vi "TPNT_LogTP.vi"(6 "UTC":bool, 7 "tpnt_logfile":path, 8 "error in (no error)":errorcluster, 9 "tp separator":string=", ", 10 "Device":T1={"device"="", "devupdate"=0.0, "next_update"=0, "devinterface"="", "TPs"=[], "Alarms"=TRUE, "monitor"=TRUE, "log sep"=""} {"TPs"."Log"."updaterate" format="%.2f"; "TPs"."Samples"."Values" format="%.2f"; "TPs"."Samples"."samples" min=1 step=1; "TPs"."Limits"."Nominal" format="%.2f"; "TPs"."Limits"."Upper" format="%.2f"; "TPs"."Limits"."Lower" format="%.2f"; "TPs"."update_rate" format="%.2f"; "devupdate" format="%.2f"}) -> (0 "error out":errorcluster, 2 "Devices out":T1={"device"="", "devupdate"=0.0, "next_update"=0, "devinterface"="", "TPs"=[], "Alarms"=TRUE, "monitor"=TRUE, "log sep"=""} {"TPs"."Log"."updaterate" format="%.2f"; "TPs"."Samples"."Values" format="%.2f"; "TPs"."Samples"."samples" min=1 step=1; "TPs"."Limits"."Nominal" format="%.2f"; "TPs"."Limits"."Upper" format="%.2f"; "TPs"."Limits"."Lower" format="%.2f"; "TPs"."update_rate" format="%.2f"; "devupdate" format="%.2f"})   [LabVIEW 2016]
uses:
  TPNT_DeviceTPs.ctl
  TPNT_TP.ctl
  TPNT_Limits.ctl
  TPNT_Samples.ctl
  TPNT_Log.ctl
panel:
  in  "maxfilesize":u32=1024
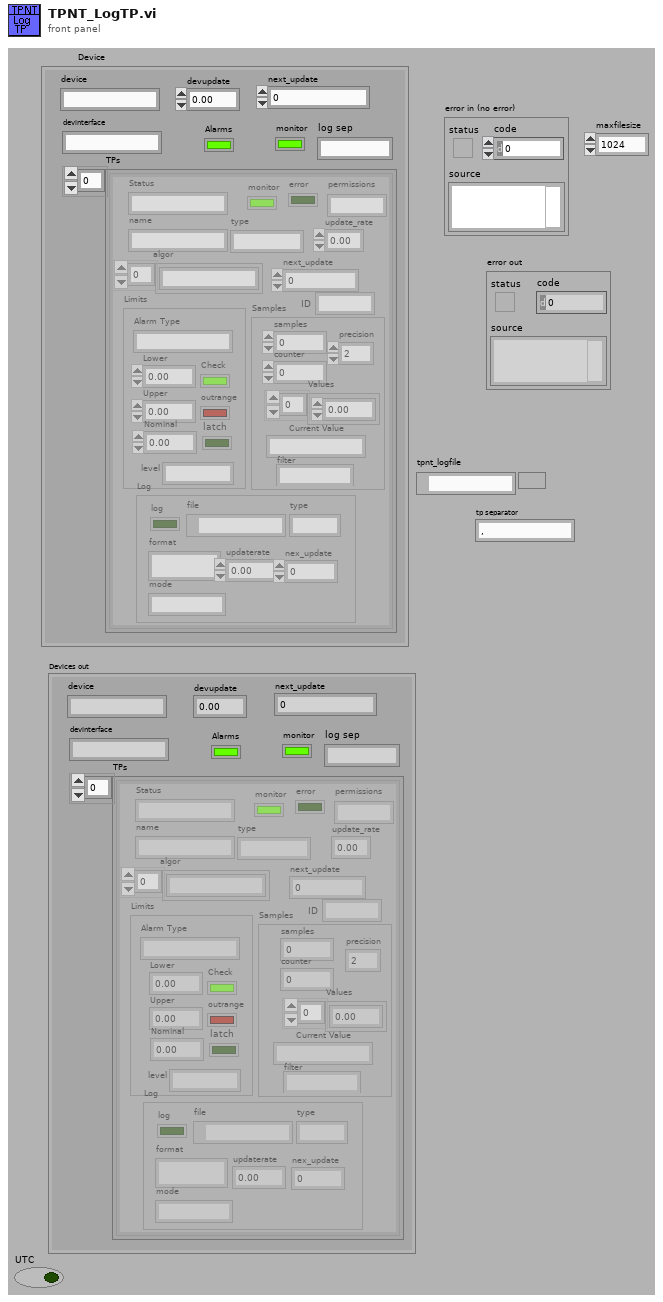
[diagram p1: front panel]
types:
  T1 = typedef "TPNT_DeviceTPs.ctl" = cluster{"device":string, "devupdate":dbl, "next_update":u32, "devinterface":string, "TPs":T2[], "Alarms":bool, "monitor":bool, "log sep":string}
  T2 = typedef "TPNT_TP.ctl" = cluster{"name":string, "type":string, "algor":string[], "update_rate":sgl, "Limits":T3, "Samples":T4, "next_update":u32, "Status":string, "monitor":bool, "error":bool, "Log":T5, "permissions":string, "ID":string}
  T3 = typedef "TPNT_Limits.ctl" = cluster{"Alarm Type":string, "Lower ":dbl, "Upper":dbl, "Nominal":dbl, "outrange":bool, "Check":bool, "latch":bool, "level":string}
  T4 = typedef "TPNT_Samples.ctl" = cluster{"samples":i32, "counter":i32, "Values":dbl[], "Current Value":string, "filter":string, "precision":u8}
  T5 = typedef "TPNT_Log.ctl" = cluster{"log":bool, "file":path, "type":string, "format":string, "updaterate":dbl, "nex_update":u32, "mode":string}
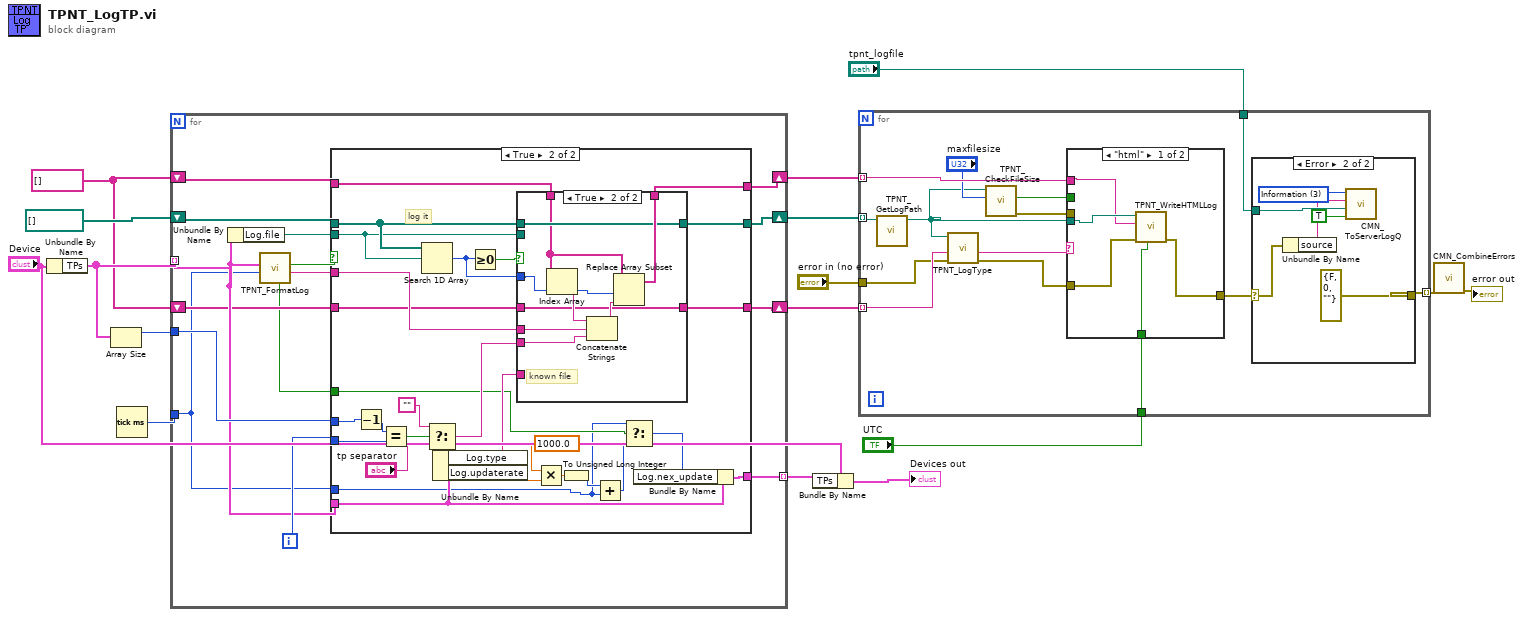
[diagram p0: block diagram]
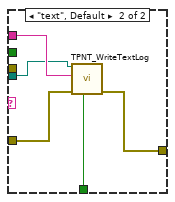
[diagram p3: hidden frame]
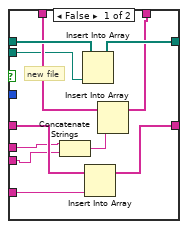
[diagram p5: hidden frame]
diagram:
  w9 = string[] []
  n1 = Unbundle By Name("Device") -> ("TPs"=w16:T2[])
  n2 = Array Size(array=w16) -> (size(s)=w10:i32)
  n3 = Tick Count (ms)() -> (millisecond timer value=w14:u32)
  n4 = for {
    tunnel: w16 -> [w22] mode=indexing
    shift-right: [w28] -> w8
    shift-left: path[] [] -> [w31]
    shift-right: [w29] -> w7
    shift-left: w9 -> [w30]
    tunnel: w14 -> [w18]
    tunnel: [w26] -> w13 mode=indexing
    tunnel: w10 -> [w25]
    shift-right: [w19] -> w6
    shift-left: w9 -> [w20]
    i -> [w27]
    n5 = Unbundle By Name(w22) -> ("Log.file"=w21:path)
    n6 = call "TPNT_FormatLog.vi"("time in"=w18, "testpoint In"=w22) -> ("message to log"=w23:string, "LOG?"=w24:bool, "by alarm"=w17:bool)  [unwired: 7 out]
    n7 = case shown="True" w24 {
      tunnel: w31 -> [w34 w44]
      tunnel: w30 -> [w35 w62]
      tunnel: [w35 w60] -> w29
      tunnel: [w34 w53] -> w28
      tunnel: w25 -> [_ w59]
      tunnel: w27 -> [_ w57]
      tunnel: w22 -> [w33 w52]
      tunnel: w18 -> [_ w38]
      tunnel: [w33 w47] -> w26
      tunnel: w23 -> [_ w46]
      tunnel: w21 -> [_ w43]
      tunnel: w20 -> [w32 w42]
      tunnel: [w32 w41] -> w19
      tunnel: w17 -> [_ w39]
      frame False {
        # "do not log, skip it"
      }
      frame True {
        # "log it"
        n8 = Decrement(x=w59) -> (x-1=w58:i32)
        n9 = Equal?(x=w58, y=w57) -> (x = y?=w56:bool)
        n10 = Search 1D Array(1D array=w44, element=w43) -> (index of element=w61:i32)  [unwired: 1 out]
        n11 = Select(t="", s=w56, f="tp separator") -> (s? t:f=w45:string)
        n12 = Unbundle By Name(w52) -> ("Log.type"=w40:string, "Log.updaterate"=w51:dbl)
        n13 = Greater Or Equal To 0?(x=w61) -> (x >= 0?=w63:bool)
        n14 = case shown="True" w63 {
          tunnel: w62 -> [w73 w78]
          tunnel: w61 -> [_ w81]
          tunnel: [w71 w83] -> w60
          tunnel: w44 -> [w74 w82]
          tunnel: [w72 w82] -> w53
          tunnel: w46 -> [w65 w77]
          tunnel: w45 -> [w66 w75]
          tunnel: w43 -> [w70 _]
          tunnel: w42 -> [w69 w76]
          tunnel: [w68 w76] -> w41
          tunnel: w40 -> [w67 _]
          frame False {
            # "new file"
            n15 = Concatenate Strings(w65, w66) -> (w64:string)
            n16 = Insert Into Array(array=w74, new element=w70) -> (w72:path[])  [unwired: 1 in]
            n17 = Insert Into Array(array=w69, new element=w67) -> (w68:string[])  [unwired: 1 in]
            n18 = Insert Into Array(array=w73, new element=w64) -> (w71:string[])  [unwired: 1 in]
          }
          frame True {
            # "known file"
            n19 = Index Array(array=w78, index=w81) -> (element=w80:string)
            n20 = Concatenate Strings(w80, w77, w75) -> (w79:string)
            n21 = Replace Array Subset(array=w78, new element=w79, index=w81) -> (w83:string[])
          }
        }
        n22 = Multiply(x=sgl 1000.0, y=w51) -> (x*y=w49:dbl)
        n23 = To Unsigned Long Integer(number=w49) -> (unsigned 32bit integer=w48:u32)
        n24 = Add(x=w48, y=w38) -> (x+y=w37:u32)
        n25 = Select(t=w38, s=w39, f=w37) -> (s? t:f=w36:u32)
        n26 = Bundle By Name(cluster=w52, "Log.nex_update"=w36) -> (w47:T2)
      }
    }
  }
  n27 = Bundle By Name(cluster="Device", "TPs"=w13) -> (→"Devices out":T1)
  n28 = for {
    tunnel: w8 -> [w85] mode=indexing
    tunnel: w7 -> [w97] mode=indexing
    tunnel: w6 -> [w96] mode=indexing
    tunnel: "error in (no error)" -> [w95]
    tunnel: [w88] -> w4 mode=indexing
    tunnel: "tpnt_logfile" -> [w87]
    tunnel: "UTC" -> [w86]
    n29 = call "TPNT_GetLogPath.vi"("logpath in"=w85) -> ("logpath out"=w84:path)  [unwired: 10 out]
    n30 = call "TPNT_LogType.vi"("error in (no error)"=w95, "type in"=w96, "File"=w84) -> ("error out"=w94:errorcluster, "type out"=w93:string)  [unwired: 7 out]
    n31 = call "TPNT_CheckFileSize.vi"("maxfilesize"="maxfilesize", "File"=w84) -> ("error out"=w91:errorcluster, "file moved"=w90:bool)  [unwired: 1 in, 7 out]
    n32 = case shown="\"html\"" w93 {
      tunnel: w97 -> [w106 w114]
      tunnel: w84 -> [w107 w113]
      tunnel: w94 -> [w109 w112]
      tunnel: [w108 w111] -> w89
      tunnel: w91 -> [_ _]
      tunnel: w90 -> [_ _]
      tunnel: w86 -> [w105 w110]
      frame "html" {
        n33 = call "TPNT_WriteHTMLLog.vi"("UTC"=w105, "error in (no error)"=w109, "message"=w106, "File"=w107) -> ("error out"=w108:errorcluster)  [unwired: 2 in, 5 out]
      }
      frame "text", Default {
        n34 = call "TPNT_WriteTextLog.vi"("UTC"=w110, "error in (no error)"=w112, "message"=w114, "File"=w113) -> ("error out"=w111:errorcluster)  [unwired: 2 in, 5 out]
      }
    }
    n35 = case shown="Error" w89 {
      selector: w89 -> [w98 w101]
      tunnel: [w98 errorcluster {"status"=FALSE, "code"=0, "source"=""} ("error IO")] -> w88
      tunnel: w87 -> [_ w103]
      frame No Error {
      }
      frame Error {
        w102 = u16 3 items=["command", "imediateReply", "Callback Reply", "Information", "none"] ("type")
        n36 = Unbundle By Name(w101) -> ("source"=w100:string)
        n37 = call "CMN_ToServerLogQ.vi"("Log"=TRUE, "file"=w103, "string"=w100, "type"=w102) -> ()  [unwired: 2 in, 5 out]
      }
    }
  }
  n38 = call "CMN_CombineErrors.vi"("Errors"=w4) -> ("error out"=→"error out":errorcluster)  [unwired: 10 out]
